vi "WriteLog.vi"(6 "FileExtension":string, 7 "MaxFileSize":i32, 8 "error in (no error)":errorcluster, 9 "Log":string, 10 "LogFolder":path, 11 "LogfileRef In":refnum<file>) -> (0 "error out":errorcluster, 3 "LogfileRef Out":refnum<file>)   [LabVIEW 2016, in "Log4Lv.lvlib"]
doc: "Use this template to build a VI to use as a subVI."
uses:
  Log4Lv.lvlib
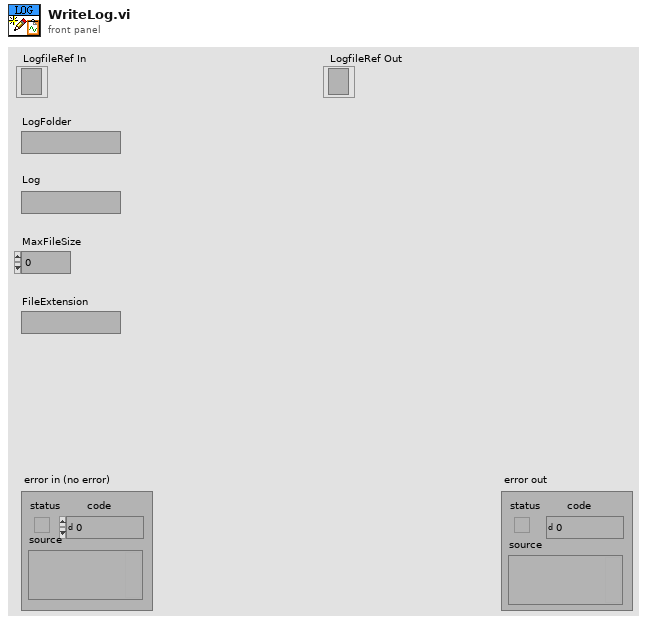
[diagram p1: front panel]
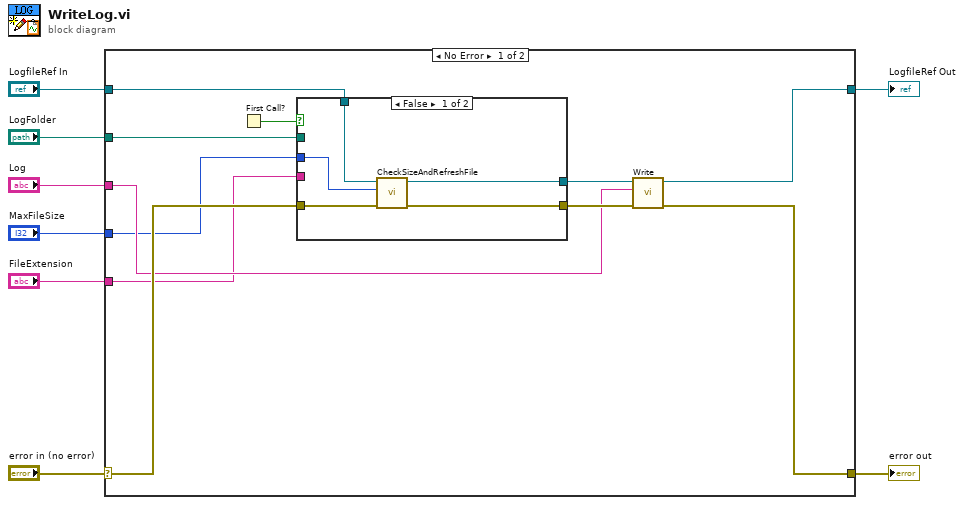
[diagram p0: block diagram]
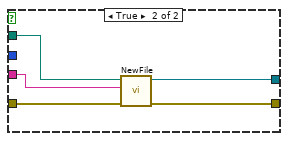
[diagram p2: hidden frame]
diagram:
  n1 = case shown="No Error" "error in (no error)" {
    selector: "error in (no error)" -> [w15 w31]
    tunnel: [w13 w31] -> w7
    tunnel: [w12 w30] -> w6
    tunnel: "LogfileRef In" -> [w18 w30]
    tunnel: "Log" -> [w14 _]
    tunnel: "LogFolder" -> [w11 _]
    tunnel: "MaxFileSize" -> [w10 _]
    tunnel: "FileExtension" -> [w9 _]
    frame No Error {
      n2 = First Call?() -> (First Call?: T/F=w19:bool)
      n3 = case shown="False" w19 {
        tunnel: w11 -> [_ w29]
        tunnel: [w21 w28] -> w17
        tunnel: w18 -> [w24 _]
        tunnel: [w22 w27] -> w16
        tunnel: w15 -> [w23 w26]
        tunnel: w10 -> [w20 _]
        tunnel: w9 -> [_ w25]
        frame False {
          n4 = call "CheckSizeAndRefreshFile.vi"("error in (no error)"=w23, "MaxFileSize"=w20, "LogfileRef In"=w24) -> ("error out"=w22:errorcluster, "LogfileRef Out"=w21:refnum<file>)  [unwired: 7 in]
        }
        frame True {
          n5 = call "NewFile.vi"("error in (no error)"=w26, "FileExtension"=w25, "LogFolder"=w29) -> ("error out"=w27:errorcluster, "LogfileRef Out"=w28:refnum<file>)  [unwired: 7 in]
        }
      }
      n6 = call "Write.vi"("Logfile Ref In"=w17, "Log"=w14, "error in (no error)"=w16) -> ("Logfile Ref Out"=w12:refnum<file>, "error out"=w13:errorcluster)  [unwired: 6 in]
    }
    frame Error {
    }
  }
  "error out" <- w7
  "LogfileRef Out" <- w6
